vi "open camera.vi"() -> ()   [LabVIEW 2018]
uses:
  <vilib>/userdefined/High Color/IMAQdx.ctl
  <vilib>/vision/driver/NI_Vision_Acquisition_Software.lvlib
  <resource>/objmgr/imaqdx.rc
panel:
  out "ty":string[](array[string])
  out "Image":T1(plugin-control)
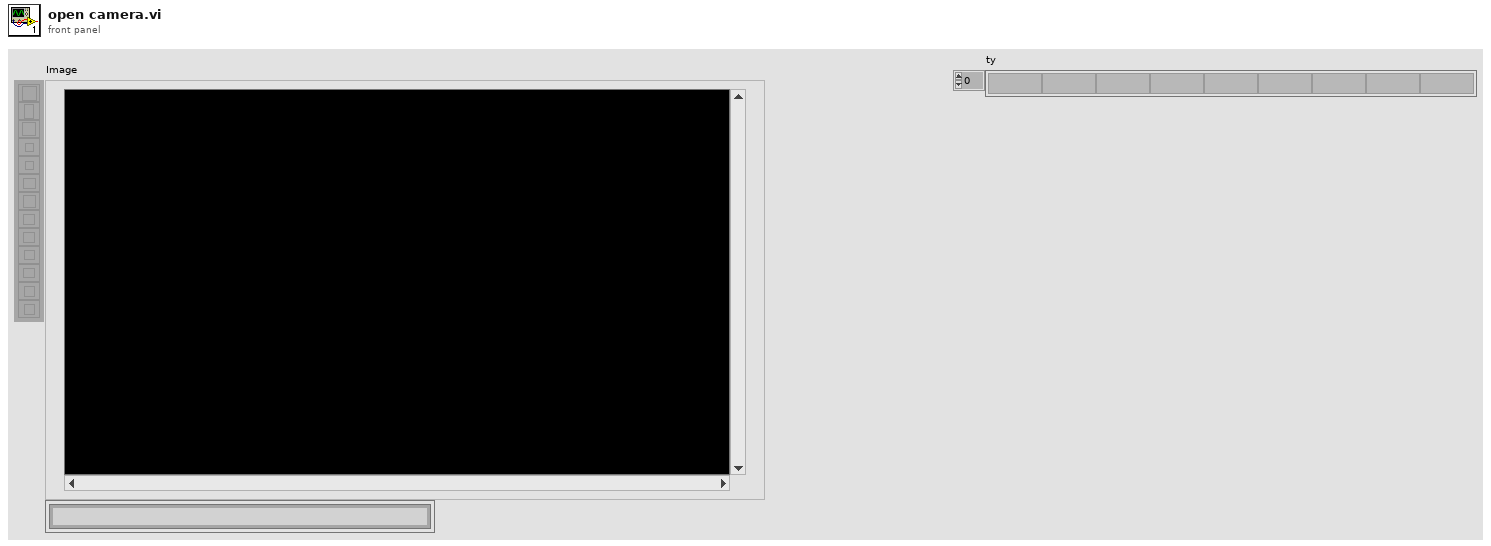
[diagram p1: front panel]
types:
  T1 = typedef "IMAQ Image.ctl" = refnum<image>
  T2 = typedef "IMAQdx.ctl" = refnum<k21>
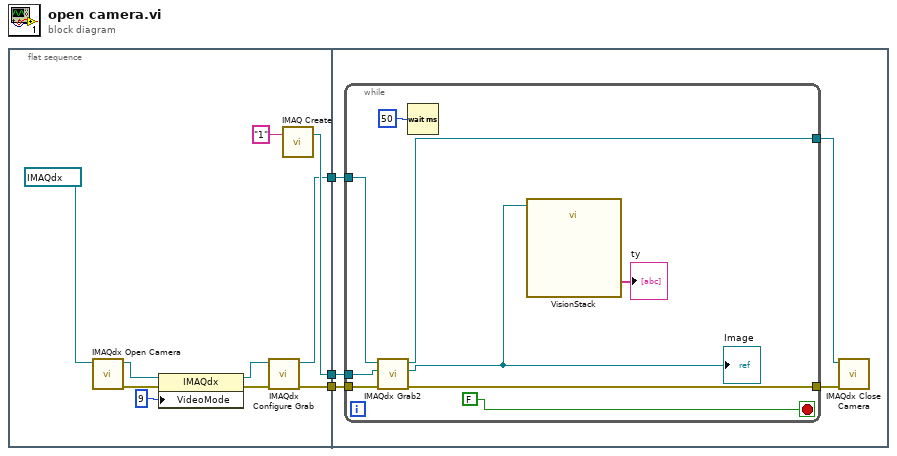
[diagram p0: block diagram]
diagram:
  n1 = flat-sequence {
    tunnel: [w6] -> w3
    tunnel: [w5] -> w2
    tunnel: [w4] -> w1
    tunnel: w3 -> [w16]
    tunnel: w2 -> [w15]
    tunnel: w1 -> [w14]
    frame #0 {
      n2 = call <vilib>:"IMAQdx Open Camera.vi"("Session In"=T2 "cam0") -> ("error out"=w11:errorcluster, "Session Out"=w10:T2)  [unwired: 9 in]
      n3 = property class="IMAQdx"(reference=w10, error in=w11, "VideoMode"=u32 9) -> (reference out=w13:T2, error out=w12:errorcluster)
      n4 = call <vilib>:"IMAQdx Configure Grab.vi"("error in"=w12, "Session In"=w13) -> ("error out"=w5:errorcluster, "Session Out"=w4:T2)  [unwired: 8 in]
      n5 = call "IMAQ Create"("Image Name"="1") -> ("New Image"=w6:T1)  [unwired: 4 in, 1 out]
    }
    frame #1 {
      n6 = while {
        tunnel: [w27] -> w18
        tunnel: [w26] -> w17
        tunnel: w16 -> [w24]
        tunnel: w15 -> [w23]
        tunnel: w14 -> [w22]
        stop <- FALSE stop-if-true
        n7 = call <vilib>:"IMAQdx Grab2.vi"("error in"=w23, "Image In"=w24, "Session In"=w22) -> ("error out"=w26:errorcluster, "Image Out"=w20:T1, "Session Out"=w27:T2)  [unwired: 5 in, 1 out]
        "Image" <- w20
        n8 = Wait (ms)(milliseconds to wait=u32 50) -> ()  [unwired: 1 out]
        n9 = call "VisionStack"("Image In"=w20) -> ("Classes (Color Classification 1)"=→"ty":string[])  [unwired: 23 in, 3 out]
      }
      n10 = call <vilib>:"IMAQdx Close Camera.vi"("error in"=w17, "Session In"=w18) -> ()  [unwired: 9 in, 1 out]
    }
  }
